vi "Update Select Module Ring.vi"(8 "error in (no error)":errorcluster, 11 "Select Module MCL Ref":refnum<vi>) -> (0 "error out":errorcluster, 3 "New Module Ring Value":i32=-1)   [LabVIEW 2014, in "Configurable.lvlib"]
doc: "Retrieve all currently running cloneable module instances and populate the module selector ring with their names and values.\n_____\nBased on Delacor QMH Project Template 4.0.0.47."
uses:
  Configurable.lvlib
  Clone Registration/Clone Registration.lvlib
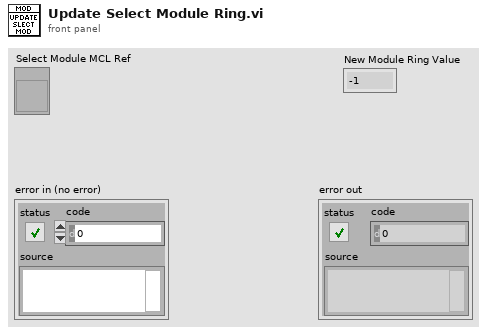
[diagram p1: front panel]
types:
  T1 = typedef "Configurable.lvlib/GetQualifiedName (Reply Payload)--cluster.ctl" = cluster{"Fully Qualified Name":string, "GetQualifiedName_error":errorcluster}
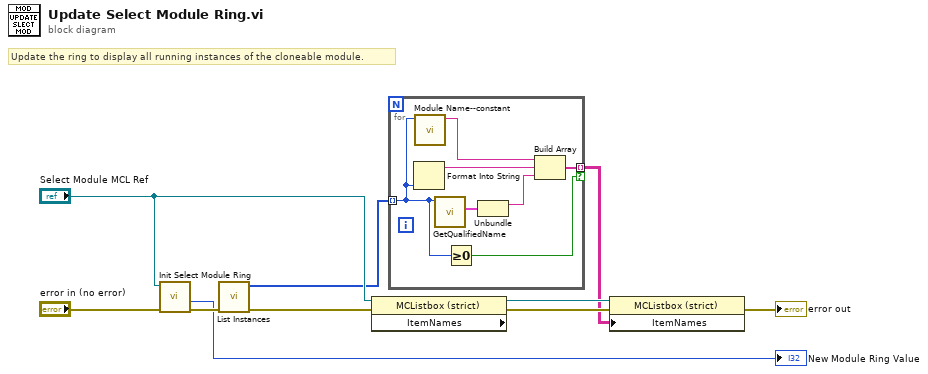
[diagram p0: block diagram]
diagram:
  # "Update the ring to display all running instances of the cloneable module."
  n1 = call "Init Select Module Ring.vi"("error in (no error)"="error in (no error)", "Select Module MCL Ref"="Select Module MCL Ref") -> ("error out"=w7:errorcluster, "Module MCL Value"=→"New Module Ring Value":i32)  [unwired: 7 in, 1 out]
  n2 = call "List Instances.vi"("error in (no error)"=w7) -> ("error out"=w1:errorcluster, "Module IDs"=w6:i32[])  [unwired: 6 in, 3 out]
  n3 = property on="Property Node" class="MCListbox (strict)" props=["ItemNames"](reference="Select Module MCL Ref", error in=w1) -> (reference out=w9:refnum<vi>, error out=w10:errorcluster)  [unwired: 1 out]
  n4 = for {
    tunnel: w6 -> [w12] mode=indexing
    tunnel: [w14] -> w2 mode=indexing if=w13
    n5 = Format Into String(w12) -> (resulting string=w17:string)  [unwired: 3 in, 1 out]
    n6 = call "Module Name--constant.vi"("Module ID"=w12) -> ("Module Name"=w11:string)  [unwired: 10 in]
    n7 = call "GetQualifiedName.vi"("Module ID"=w12) -> ("Reply Payload"=w16:T1)  [unwired: 8 in, 2 out]
    n8 = Greater Or Equal To 0?(x=w12) -> (x >= 0?=w13:bool)
    n9 = Unbundle(w16) -> ("Fully Qualified Name"=w15:string)  [unwired: 1 out]
    n10 = Build Array(w11, w17, w15) -> (w14:string[])
  }
  n11 = property on="Property Node" class="MCListbox (strict)"(reference=w9, error in=w10, "ItemNames"=w2) -> (error out=→"error out":errorcluster)  [unwired: 1 out]
